vi "Client-全局变量.vi"() -> ()   [LabVIEW 2013]
panel:
  out "本机IP":string
  out "设备-配置侦听TCP-Port":u16=61000
  out "云服务连接信息":T1
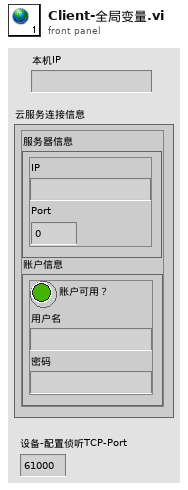
[diagram p1: front panel]
types:
  T1 = cluster{"服务器信息":cluster{"IP":string, "Port":u16}, "账户信息":cluster{"账户可用？":bool, "用户名":string, "密码":string}}
diagram:
